vi "Filter FPGA by Device Code.vi"(8 "error in (no error)":errorcluster, 10 "Device Code":string, 11 "FPGA Personality File Paths":path[](array[path])) -> (0 "error out":errorcluster, 3 "Filtered FPGA Personality File Paths":path[](array[path]))   [LabVIEW 2021, in "Personality.lvlib"]
doc: "Filters the FPGA personality paths with specified device code."
uses:
  <vilib>/myRIO/Common/FPGA Personality Framework/Personality.lvlib
  <vilib>/xml/Load XML File.vi
  <vilib>/xml/Close Reference(Node).vi
  <vilib>/xml/NI_XML.lvlib
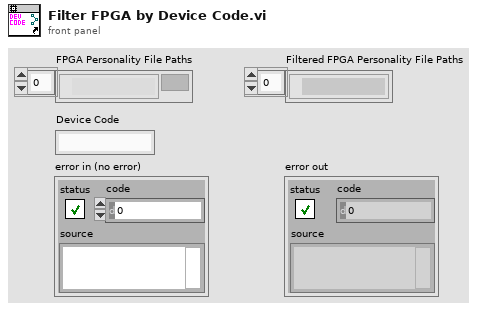
[diagram p1: front panel]
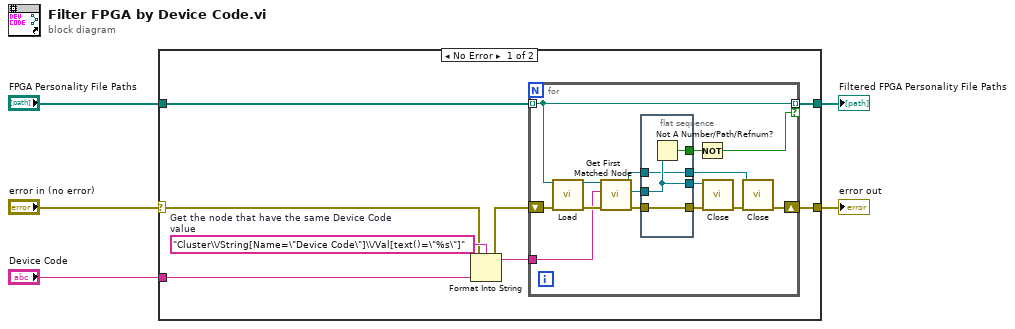
[diagram p0: block diagram]
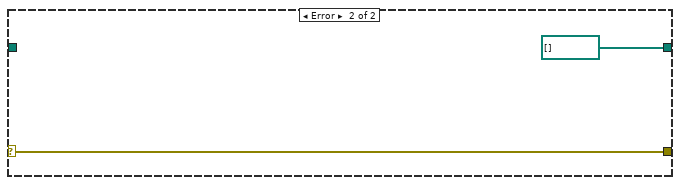
[diagram p2: hidden frame]
diagram:
  n1 = case shown="No Error" "error in (no error)" {
    selector: "error in (no error)" -> [w8 w34]
    tunnel: "FPGA Personality File Paths" -> [w11 _]
    tunnel: [w10 w34] -> w4
    tunnel: [w9 path[] []] -> w3
    tunnel: "Device Code" -> [w6 _]
    frame No Error {
      w13 = "Cluster\\/String[Name=\"Device Code\"]\\/Val[text()=\"%s\"]"  # Get the node that have the same Device Code value
      n2 = Format Into String(format string=w13, error in=w8, w6) -> (resulting string=w12:string, error out=w7:errorcluster)  [unwired: 1 in]
      n3 = for {
        shift-right: [w21] -> w10
        shift-left: w7 -> [w27]
        tunnel: w11 -> [w23] mode=indexing
        tunnel: w12 -> [w24]
        tunnel: [w23] -> w9 mode=indexing if=w22
        n4 = call-poly <vilib>:"Load.vi"("path to XML document"=w23, "error in (no error)"=w27) -> ("DOM document out"=w28:refnum<k20>, "error out"=w26:errorcluster)  [unwired: 11 in, 1 out]
        n5 = call <vilib>:"Get First Matched Node.vi"("error in (no error)"=w26, "XPath expression"=w24, "node in"=w28) -> ("error out"=w20:errorcluster, "node result"=w19:refnum<k20>, "node out"=w15:refnum<k20>)  [unwired: 6 in]
        n6 = flat-sequence {
          tunnel: [w32] -> w16
          tunnel: w20 -> [w30]
          tunnel: w19 -> [w31]
          tunnel: [w31] -> w18
          tunnel: [w30] -> w17
          tunnel: w15 -> [w29]
          tunnel: [w29] -> w14
          frame #0 {
            n7 = Not A Number/Path/Refnum?(number/path/refnum=w31) -> (NaN/Path/Refnum?=w32:bool)
          }
        }
        n8 = Not(x=w16) -> (.not. x?=w22:bool)
        n9 = call-poly <vilib>:"Close.vi"("error in (no error)"=w17, "node"=w18) -> ("error out"=w25:errorcluster)  [unwired: 7 in]
        n10 = call-poly <vilib>:"Close.vi"("error in (no error)"=w25, "node"=w14) -> ("error out"=w21:errorcluster)  [unwired: 7 in]
      }
    }
    frame Error {
    }
  }
  "Filtered FPGA Personality File Paths" <- w3
  "error out" <- w4
